vi "UI Message Loop.vi"(8 "error in (no error)":errorcluster, 11 "UI Queue In":refnum<queue>) -> (0 "error out":errorcluster, 3 "UI Queue Out":refnum<queue>)   [LabVIEW 2016]
uses:
  Controls/Message Structure.ctl
  Classes/Lamp/Container/Lamp Container.lvclass
  Controls/Operational Modes.ctl
  Controls/Lamps Manual.ctl
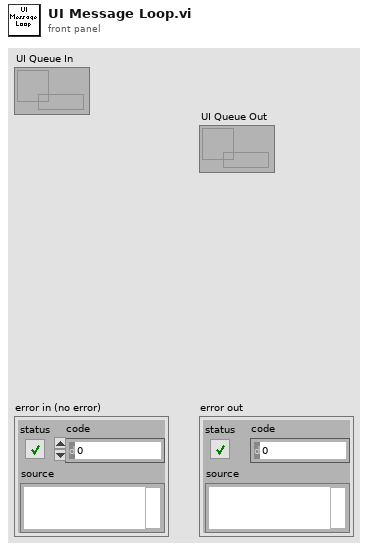
[diagram p1: front panel]
types:
  T1 = typedef "Operational Modes.ctl" = enum16{"Sci", "Sci-LFC", "Solar", "Solar-LFC", "LFC", "LFC-Sim", "LFC-Both", "ThAr", "ThAr-LFC", "Flat", "ExtFlat", "ExtFlat-Sim", "ExtFlat-Both", "Qtz", "ExtQtz", "ExtQtz-Sim", "ExtQtz-Both", "Dark", "Manual", "Off"}
  T2 = typedef "Lamps Manual.ctl" = cluster{"ThAr":bool, "Quartz":bool, "LED":bool, "ThAr Timeout":dbl, "LED Timeout":dbl, "Quartz Timeout":dbl}
  T3 = typedef "Lamps.ctl" = cluster{"ThAr":cluster{"Time Stamp":timestamp, "Status":bool, "Timeout":dbl}, "LED":cluster{"Time Stamp":timestamp, "Status":bool, "Timeout":dbl}, "Quartz":cluster{"Time Stamp":timestamp, "Status":bool, "Timeout":dbl}}
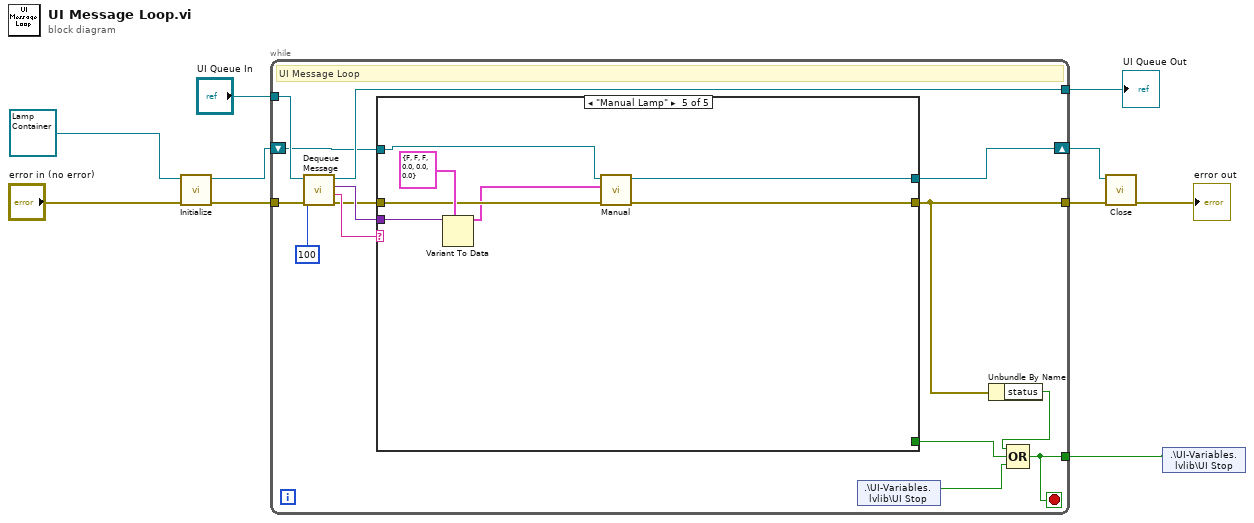
[diagram p0: block diagram]
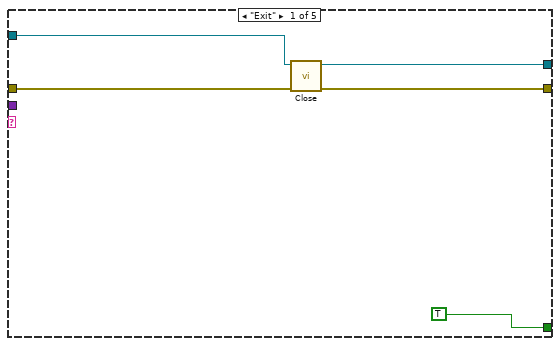
[diagram p2: hidden frame]
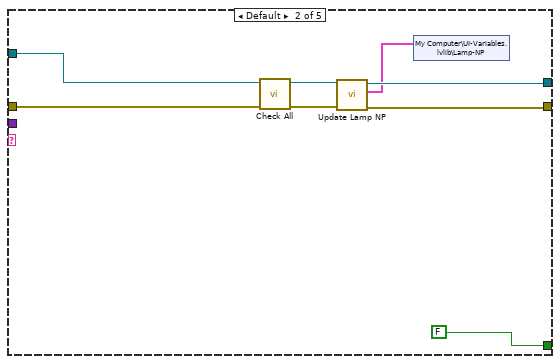
[diagram p3: hidden frame]
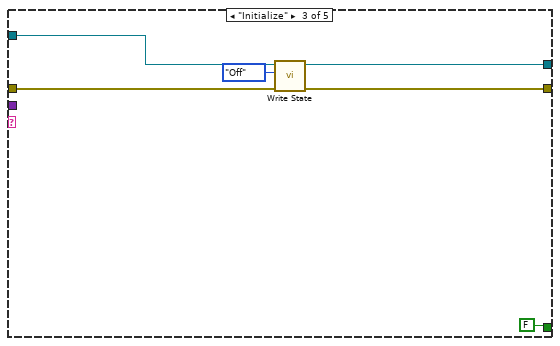
[diagram p4: hidden frame]
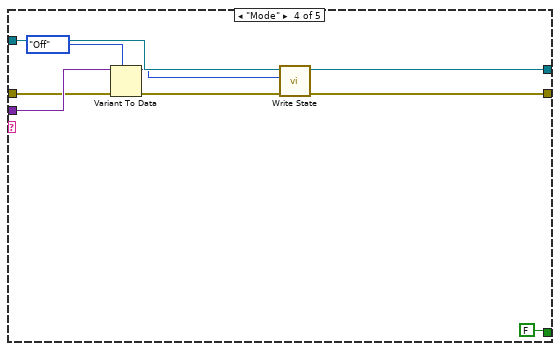
[diagram p5: hidden frame]
diagram:
  n1 = call-dynamic "Initialize.vi"("error in (no error)"="error in (no error)", "Lamp Container in"=refnum<class "Lamp Container.lvclass"> refnum ("Lamp Container.lvclass")) -> ("error out"=w5:errorcluster, "Lamp Container out"=w4:refnum<class "Lamp Container.lvclass">)  [unwired: 8 in]
  n2 = while {
    tunnel: "UI Queue In" -> [w18]
    tunnel: [w20] -> w3
    tunnel: w5 -> [w19]
    tunnel: [w14] -> w9
    tunnel: [w22] -> w8
    shift-right: [w11] -> w1
    shift-left: w4 -> [w12]
    stop <- w22 stop-if-true
    # "UI Message Loop"
    n3 = call "Dequeue Message.vi"("error in (no error)"=w19, "timeout in ms (-1)"=100, "Queue in"=w18) -> ("error out"=w15:errorcluster, "Cmd"=w17:string, "Data"=w16:variant, "Queue out"=w14:refnum<queue>)  [unwired: 5 in]
    n4 = case shown="\"Manual Lamp\"" w17 {
      tunnel: [TRUE FALSE FALSE FALSE _] -> w24
      tunnel: w16 -> [_ _ _ w52 w59]
      tunnel: w15 -> [w28 w35 w41 w50 w55]
      tunnel: [w27 w33 w40 w46 w56] -> w20
      tunnel: w12 -> [w25 w36 w43 w49 w54]
      tunnel: [w26 w32 w39 w48 w57] -> w11
      frame "Exit" {
        n5 = call-dynamic "Close.vi"("error in (no error)"=w28, "Lamp Container in"=w25) -> ("error out"=w27:errorcluster, "Lamp Container out"=w26:refnum<class "Lamp Container.lvclass">)  [unwired: 8 in]
      }
      frame Default {
        n6 = call-dynamic "Check All.vi"("error in (no error)"=w35, "Lamp Container in"=w36) -> ("error out"=w34:errorcluster, "Lamp Container out"=w31:refnum<class "Lamp Container.lvclass">)  [unwired: 8 in]
        n7 = call "Update Lamp NP.vi"("error in (no error)"=w34, "Lamp Container In"=w31) -> ("error out"=w33:errorcluster, "Lamps"=w30:T3, "Lamp Container Out"=w32:refnum<class "Lamp Container.lvclass">)  [unwired: 7 in]
        n8 = shared-variable "My Computer\\UI-Variables.lvlib\\Lamp-NP"(w30) -> ()  [unwired: 1 in, 1 out]
      }
      frame "Initialize" {
        n9 = call-dynamic "Write State.vi"("error in (no error)"=w41, "OpMode"=Operational_Modes."Off", "Lamp Container in"=w43) -> ("error out"=w40:errorcluster, "Lamp Container out"=w39:refnum<class "Lamp Container.lvclass">)  [unwired: 7 in]
      }
      frame "Mode" {
        n10 = Variant To Data(error in=w50, type=Operational_Modes."Off" ("EXPRES Mode 2"), Variant=w52) -> (data=w45:T1, error out=w47:errorcluster)
        n11 = call-dynamic "Write State.vi"("error in (no error)"=w47, "OpMode"=w45, "Lamp Container in"=w49) -> ("error out"=w46:errorcluster, "Lamp Container out"=w48:refnum<class "Lamp Container.lvclass">)  [unwired: 7 in]
      }
      frame "Manual Lamp" {
        n12 = Variant To Data(type=T2 {"ThAr"=FALSE, "Quartz"=FALSE, "LED"=FALSE, "ThAr Timeout"=0.0, "LED Timeout"=0.0, "Quartz Timeout"=0.0} ("Manual Lamp"), Variant=w59) -> (data=w53:T2)  [unwired: 1 in, 1 out]
        n13 = call-dynamic "Manual.vi"("error in (no error)"=w55, "Manual Lamp"=w53, "Lamp Container in"=w54) -> ("error out"=w56:errorcluster, "Lamp Container out"=w57:refnum<class "Lamp Container.lvclass">)  [unwired: 7 in]
      }
    }
    n14 = shared-variable ".\\UI-Variables.lvlib\\UI Stop"() -> (w23:bool)  [unwired: 1 in, 1 out]
    n15 = Unbundle By Name(w20) -> ("status"=w21:bool)
    n16 = Compound Arithmetic op=OR(w21, w24, w23) -> (w22:bool)
  }
  "UI Queue Out" <- w9
  n17 = call-dynamic "Close.vi"("error in (no error)"=w3, "Lamp Container in"=w1) -> ("error out"=→"error out":errorcluster)  [unwired: 8 in, 1 out]
  n18 = shared-variable ".\\UI-Variables.lvlib\\UI Stop"(w8) -> ()  [unwired: 1 in, 1 out]
